vi "Set Auto Open Reports.vi"(8 "error in (no error)":errorcluster, 10 "Open Generated Reports?":bool, 11 "Report In":refnum<class "Report.lvclass">) -> (0 "error out":errorcluster, 3 "Report Out":refnum<class "Report.lvclass">)   [LabVIEW 2020, in "Reports.lvlib" / "Report.lvclass"]
uses:
  Report.lvclass
  Report.lvclass/Report.ctl
  User Interface/Process/Process.lvclass/Process.ctl
  User Interface/Process/Protected/Messaging/Enqueue Message.vi
  Report Generator/Report Generator.lvclass
  C:/git/astemes-lunit/source/User Interface/Process/Process.lvclass
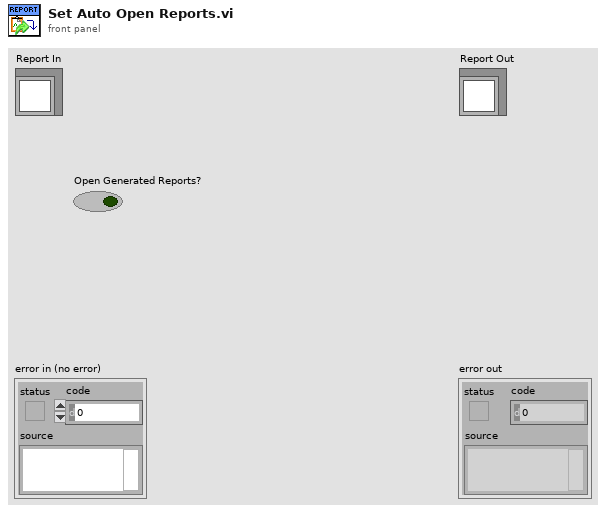
[diagram p1: front panel]
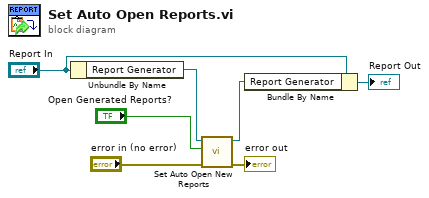
[diagram p0: block diagram]
diagram:
  n1 = Unbundle By Name("Report In") -> ("Report Generator"=w6:refnum<class "Report Generator.lvclass">)
  n2 = call "Set Auto Open New Reports.vi"("error in (no error)"="error in (no error)", "Open New Reports?"="Open Generated Reports?", "Report Generator In"=w6) -> ("error out"=→"error out":errorcluster, "Report Generator Out"=w1:refnum<class "Report Generator.lvclass">)  [unwired: 7 in]
  n3 = Bundle By Name(cluster="Report In", "Report Generator"=w1) -> (→"Report Out":refnum<class "Report.lvclass">)
